vi "QR_registro_testcompleto.vi"() -> ()   [LabVIEW 2019]
uses:
  <vilib>/Instr/_visa.llb/VISA Configure Serial Port (Instr).vi
  <vilib>/regexp/Match Regular Expression.xnode
panel:
  in  "?":bool
  out "Boolean":bool
  in  "Cerrar socket":bool
  in  "Abrir socket":bool
  out "Error_QR":bool
  in  "Interruptor Error":bool
  in  "stop socket 2":bool
  out "Bytes at port 3":u32=1
  in  "IN y":string(combo)="00"
  in  "IN x":string(combo)="00"
  in  "NOK y":string(combo)="00"
  in  "NOK x":string(combo)="00"
  in  "OK y":string(combo)="00"
  in  "OK x":string(combo)="00"
  in  "Operator's name":string(combo)="Juan Rodríguez"
  in  "?":bool
  in  "Fichero de registro":path=path "C:/Trabajo_Robot/desde Marzo 2023/Pruebas_PC_APD/RESULT_TEST_C_LABP0"
  in  "Config File":path=path "C:/Trabajo/Test Asic Javi_2021/Origen Socket SERVO_PCB_BUENO_v5 (muchos asics)/CONFIG/configuracion_robot_CTAV2022A.test"
  in  "Path Out Report":path=path "C:/Trabajo_Robot/desde Marzo 2023/Pruebas_PC_APD/RESULT_TEST_C_LABP0"
  out "Datos_QR":string
  in  "stop socket":bool
  out "Bytes at port 1":u32
  in  "Enviar":bool
  out "Iteraciones":i32=1
  out "Lectura buffer":string="1"
  in  "Delay (ms)":dbl=1.0 min=1.0 max=9.0 step=1.0
  out "Bytes at port 2":u32=1
  out "message":string=" INSTRUCTIONS:\r\rNormal Use:  When using subVIs that incorporate the error in/error out (or error I/O) structure, place this handler where you want to inform the user of an error, typically at the end of the I/O data path, as the last action of the program.  If the error in error? is ERROR, the handler creates a message describing the error and its source.  If the type of dialog = 1 (default), the message is displayed to the user, who can only acknowedge it.  If the type = 2, the user can acknowledge the message or abort execution; aborting a program with active I/O is not recommended.  If the type = 0, no message is displayed; this is used to process the error programmatically, and the error out cluster elements are wired to individual terminals for that reason.  \r\rOther Use:\n\r\nlocal testing.  To test the error code of a subVI or function that does not have the error I/O structure, you can wire its error code and a source string to the local error code and error source inputs.  If error in error? indicates no error and error code is not equal to 0, the local code and source are substituted for the error in values, and error? is set TRUE (ERROR)."
  in  "Interruptor":bool
  in  "stop":bool
  # "Funcionamiento: en la primera iteración, el efector se desplaza desde el origen hasta la celda\nintroducida, hace una pausa, va a la posición del socket (0,0), hace otra pausa, va a la celda\nde salida y vuelve al origen. En las iteraciones siguientes hará lo mismo pero recorriendo las\nceldas de la bandeja sucesivamente. Que el desplazamiento se produzca hacia una celda de\nla bandeja OK o de la bandeja NOK depende de la salidad del programa de test de Asics."
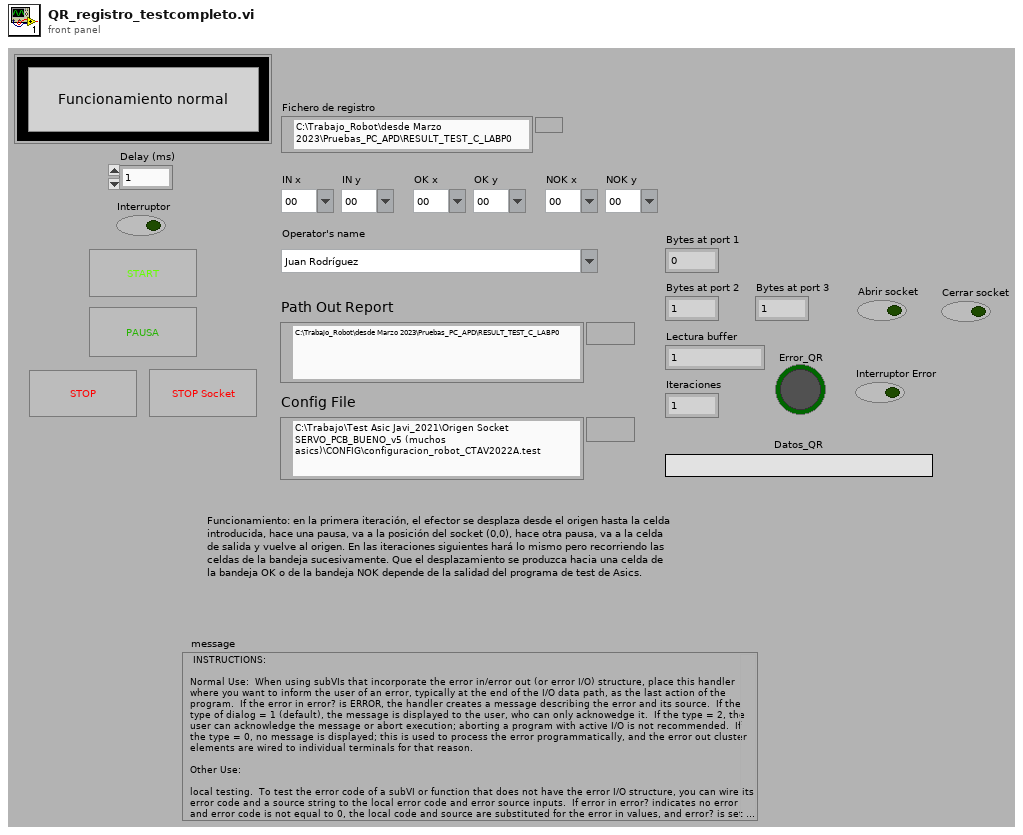
[diagram p1: front panel]
types:
  T1 = enum16{"open", "replace", "create", "open or create", "replace or create", "replace or create with confirmation"}
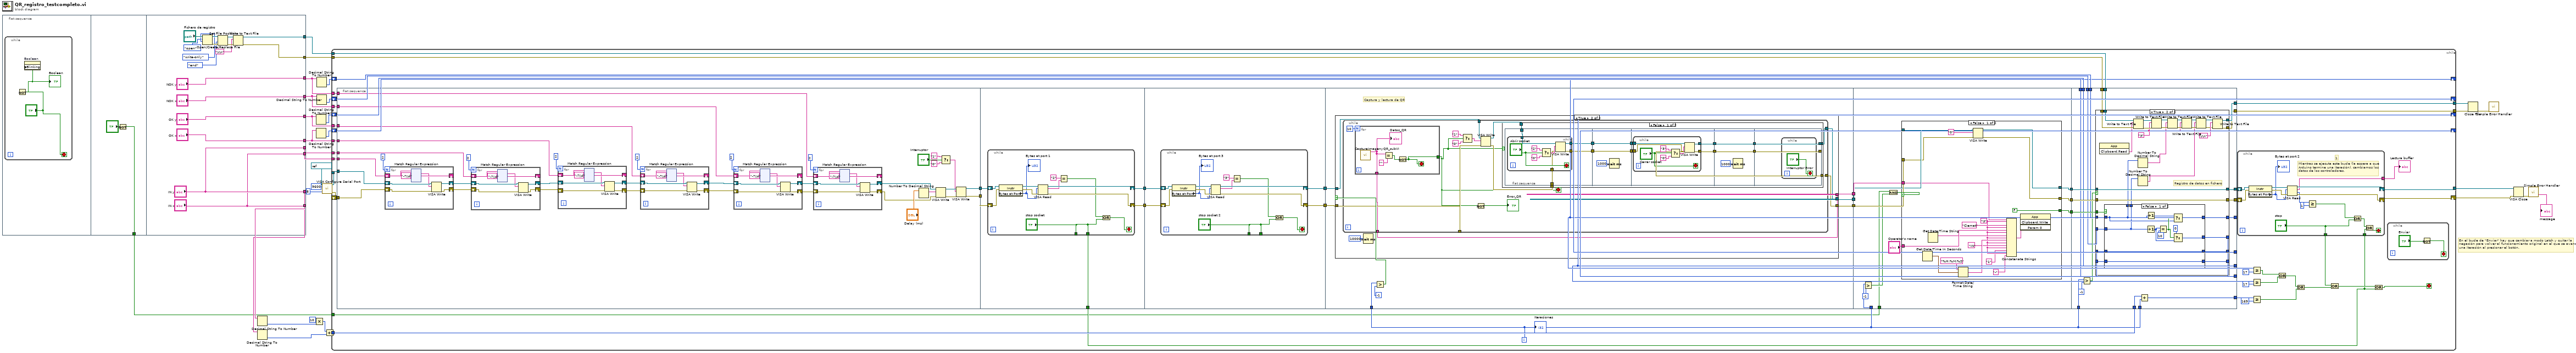
[diagram p0: block diagram]
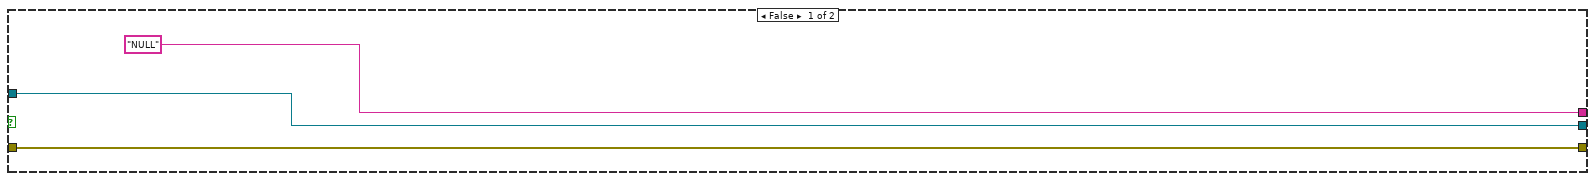
[diagram p2: hidden frame]
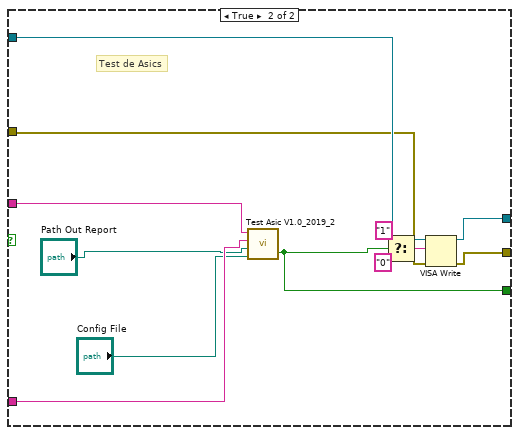
[diagram p4: hidden frame]
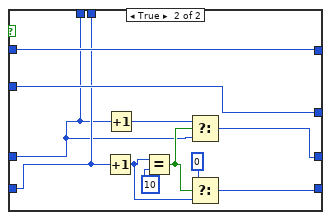
[diagram p6: hidden frame]
diagram:
  # "En el bucle de \"Enviar\" hay que cambiar a modo Latch y quitar la\nnegación para volver al funcionamiento original en el que se avanza\nuna iteración al presionar el botón."
  n1 = flat-sequence {
    tunnel: [w35] -> w1
    tunnel: ["NOK y"] -> w16
    tunnel: ["NOK x"] -> w15
    tunnel: ["OK y"] -> w14
    tunnel: ["OK x"] -> w13
    tunnel: ["IN y"] -> w12
    tunnel: ["IN x"] -> w11
    tunnel: [w37] -> w10
    tunnel: [w38] -> w9
    tunnel: ["IN y"] -> w8
    tunnel: ["IN x"] -> w7
    frame #0 {
      n2 = while {
        stop <- "?" stop-if-true
        n3 = Not(x="?") -> (.not. x?=w33:bool)
        "Boolean" <- w33
        n4 = property on="Boolean" class="Bool (strict)"("Blinking"=w33) -> ()  [unwired: 2 in, 2 out]
      }
    }
    frame #1 {
      n5 = Not(x="?") -> (.not. x?=w35:bool)
    }
    frame #2 {
      n6 = Open/Create/Replace File(file path (use dialog)="Fichero de registro", operation (0:open)=T1."open", access (0:read/write)=enum16{"read/write", "read-only", "write-only"}."write-only") -> (refnum out=w49:refnum<file>, error out=w52:errorcluster)  [unwired: 3 in, 1 out]
      n7 = Set File Position(refnum=w49, from (0:start)=enum16{"start", "end", "current"}."end", error in=w52) -> (refnum out=w50:refnum<file>, error out=w53:errorcluster)  [unwired: 1 in]
      n8 = Write to Text File(file (use dialog)=w50, text="\r\n", error in=w53) -> (refnum out=w38:refnum<file>, error out=w37:errorcluster)  [unwired: 1 in, 1 out]
    }
  }
  n9 = Decimal String To Number(string=w8) -> (number=w6:i32)  [unwired: 2 in, 1 out]
  n10 = Decimal String To Number(string=w7) -> (number=w3:i32)  [unwired: 2 in, 1 out]
  n11 = Multiply(x=10, y=w6) -> (x*y=w4:i32)
  n12 = Decimal String To Number(string=w14) -> (number=w18:i32)  [unwired: 2 in, 1 out]
  n13 = Decimal String To Number(string=w13) -> (number=w17:i32)  [unwired: 2 in, 1 out]
  n14 = Decimal String To Number(string=w16) -> (number=w20:i32)  [unwired: 2 in, 1 out]
  n15 = Decimal String To Number(string=w15) -> (number=w19:i32)  [unwired: 2 in, 1 out]
  n16 = call-poly "VISA Configure Serial Port"("VISA resource name"=refnum<visa-resource-name> "COM9", "baud rate (9600)"=u32 9600, "data bits (8)"=u16 8) -> ("VISA resource name out"=w24:refnum<visa-resource-name>, "error out"=w27:errorcluster)  [unwired: 11 in]
  n17 = Add(x=w4, y=w3) -> (x+y=w2:i32)
  n18 = while {
    shift-right: [w104] -> w25
    shift-left: w27 -> [w106]
    tunnel: w24 -> [w102]
    tunnel: [w105] -> w26
    tunnel: w9 -> [w95]
    tunnel: [w94] -> w23
    tunnel: w10 -> [w93]
    tunnel: [w92] -> w22
    tunnel: w11 -> [w90]
    tunnel: w12 -> [w89]
    tunnel: w13 -> [w88]
    tunnel: w14 -> [w87]
    tunnel: w15 -> [w86]
    tunnel: w16 -> [w85]
    shift-right: [w78] -> _
    shift-left: w20 -> [w84]
    shift-right: [w80] -> _
    shift-left: w19 -> [w83]
    shift-right: [w76] -> _
    shift-left: w18 -> [w82]
    shift-right: [w79] -> _
    shift-left: w17 -> [w81]
    tunnel: w2 -> [w72]
    tunnel: w1 -> [w54]
    i -> [w55]
    stop <- w64 stop-if-true
    n19 = flat-sequence {
      tunnel: w106 -> [w142]
      tunnel: w102 -> [w131]
      tunnel: [w133] -> w101
      tunnel: [w132] -> w100
      tunnel: w90 -> [w112]
      tunnel: w89 -> [w111]
      tunnel: w88 -> [w110]
      tunnel: w87 -> [w109]
      tunnel: w86 -> [w108]
      tunnel: w85 -> [w107]
      tunnel: w101 -> [w879]
      tunnel: w100 -> [w878]
      tunnel: [w877] -> w62
      tunnel: [w876] -> w60
      tunnel: [w875] -> w63
      tunnel: w62 -> [w895]
      tunnel: [w893] -> w61
      tunnel: w60 -> [w894]
      tunnel: [w892] -> w59
      tunnel: w61 -> [w913]
      tunnel: w59 -> [w912]
      tunnel: w55 -> [w914]
      tunnel: [w910] -> w58
      tunnel: [w909] -> w57
      tunnel: [w908] -> w56
      tunnel: w55 -> [w998]
      tunnel: [w1000] -> w98
      tunnel: [w999] -> w97
      tunnel: [w996] -> w91
      tunnel: w58 -> [w995]
      tunnel: w57 -> [w994]
      tunnel: w56 -> [w993]
      tunnel: w54 -> [w990]
      tunnel: [w1047] -> w96
      tunnel: [w1049] -> w99
      tunnel: w98 -> [w1048]
      tunnel: w97 -> [w1046]
      tunnel: w95 -> [w1053]
      tunnel: [w1052] -> w94
      tunnel: w93 -> [w1051]
      tunnel: [w1050] -> w92
      tunnel: w55 -> [w1043]
      tunnel: w91 -> [w1042]
      tunnel: w84 -> [w1038]
      tunnel: w83 -> [w1041]
      tunnel: w82 -> [w1040]
      tunnel: w81 -> [w1039]
      tunnel: [w1037] -> w78
      tunnel: [w1036] -> w80
      tunnel: [w1035] -> w76
      tunnel: [w1034] -> w79
      tunnel: w72 -> [w1033]
      tunnel: w55 -> [w1032]
      tunnel: [w1031] -> w71
      frame #0 {
        n20 = for {
          N: 2 -> [_]
          shift-right: [w754] -> _
          shift-left: w112 -> [w759]
          shift-right: [w757] -> w128
          shift-left: w131 -> [w758]
          shift-right: [w755] -> w127
          shift-left: w142 -> [w756]
          n21 = xnode "Match Regular Expression"("input string"=w759, "regular expression"="-?\\d") -> ("whole match"=w753:string, "after match"=w754:string)  [unwired: 4 in, 3 out]
          n22 = VISA Write(VISA resource name=w758, write buffer=w753, error in (no error)=w756) -> (VISA resource name out=w757:refnum<visa-resource-name>, error out=w755:errorcluster)  [unwired: 1 out]
        }
        n23 = for {
          N: 2 -> [_]
          shift-right: [w632] -> _
          shift-left: w111 -> [w637]
          shift-right: [w635] -> w122
          shift-left: w128 -> [w636]
          shift-right: [w633] -> w121
          shift-left: w127 -> [w634]
          n24 = xnode "Match Regular Expression"("input string"=w637, "regular expression"="-?\\d") -> ("whole match"=w631:string, "after match"=w632:string)  [unwired: 4 in, 3 out]
          n25 = VISA Write(VISA resource name=w636, write buffer=w631, error in (no error)=w634) -> (VISA resource name out=w635:refnum<visa-resource-name>, error out=w633:errorcluster)  [unwired: 1 out]
        }
        n26 = for {
          N: 2 -> [_]
          shift-right: [w510] -> _
          shift-left: w110 -> [w515]
          shift-right: [w513] -> w124
          shift-left: w122 -> [w514]
          shift-right: [w511] -> w123
          shift-left: w121 -> [w512]
          n27 = xnode "Match Regular Expression"("input string"=w515, "regular expression"="-?\\d") -> ("whole match"=w509:string, "after match"=w510:string)  [unwired: 4 in, 3 out]
          n28 = VISA Write(VISA resource name=w514, write buffer=w509, error in (no error)=w512) -> (VISA resource name out=w513:refnum<visa-resource-name>, error out=w511:errorcluster)  [unwired: 1 out]
        }
        n29 = for {
          N: 2 -> [_]
          shift-right: [w388] -> _
          shift-left: w109 -> [w393]
          shift-right: [w391] -> w116
          shift-left: w124 -> [w392]
          shift-right: [w389] -> w115
          shift-left: w123 -> [w390]
          n30 = xnode "Match Regular Expression"("input string"=w393, "regular expression"="-?\\d") -> ("whole match"=w387:string, "after match"=w388:string)  [unwired: 4 in, 3 out]
          n31 = VISA Write(VISA resource name=w392, write buffer=w387, error in (no error)=w390) -> (VISA resource name out=w391:refnum<visa-resource-name>, error out=w389:errorcluster)  [unwired: 1 out]
        }
        n32 = for {
          N: 2 -> [_]
          shift-right: [w266] -> _
          shift-left: w108 -> [w271]
          shift-right: [w269] -> w118
          shift-left: w116 -> [w270]
          shift-right: [w267] -> w117
          shift-left: w115 -> [w268]
          n33 = xnode "Match Regular Expression"("input string"=w271, "regular expression"="-?\\d") -> ("whole match"=w265:string, "after match"=w266:string)  [unwired: 4 in, 3 out]
          n34 = VISA Write(VISA resource name=w270, write buffer=w265, error in (no error)=w268) -> (VISA resource name out=w269:refnum<visa-resource-name>, error out=w267:errorcluster)  [unwired: 1 out]
        }
        n35 = for {
          N: 2 -> [_]
          shift-right: [w144] -> _
          shift-left: w107 -> [w149]
          shift-right: [w147] -> w114
          shift-left: w118 -> [w148]
          shift-right: [w145] -> w113
          shift-left: w117 -> [w146]
          n36 = xnode "Match Regular Expression"("input string"=w149, "regular expression"="-?\\d") -> ("whole match"=w143:string, "after match"=w144:string)  [unwired: 4 in, 3 out]
          n37 = VISA Write(VISA resource name=w148, write buffer=w143, error in (no error)=w146) -> (VISA resource name out=w147:refnum<visa-resource-name>, error out=w145:errorcluster)  [unwired: 1 out]
        }
        n38 = Number To Decimal String(number="Delay (ms)") -> (decimal integer string=w136:string)  [unwired: 1 in]
        n39 = VISA Write(VISA resource name=w114, write buffer=w136, error in (no error)=w113) -> (VISA resource name out=w138:refnum<visa-resource-name>, error out=w137:errorcluster)  [unwired: 1 out]
        n40 = Select(t="1" ("write buffer"), s="Interruptor", f="0" ("write buffer")) -> (s? t:f=w134:string)
        n41 = VISA Write(VISA resource name=w138, write buffer=w134, error in (no error)=w137) -> (VISA resource name out=w133:refnum<visa-resource-name>, error out=w132:errorcluster)  [unwired: 1 out]
      }
      frame #1 {
        n42 = while {
          shift-right: [w885] -> w876
          shift-left: w878 -> [w890]
          tunnel: ["stop socket"] -> _
          shift-right: [w886] -> w877
          shift-left: w879 -> [w891]
          tunnel: ["stop socket"] -> w875
          stop <- w881 stop-if-true
          n43 = property class="Instr"(reference=w891, error in=w890) -> (reference out=w889:refnum<visa-resource-name>, error out=w888:errorcluster, "Bytes at Port"=w887:u32)
          "Bytes at port 1" <- w887
          n44 = VISA Read(VISA resource name=w889, byte count=w887, error in (no error)=w888) -> (VISA resource name out=w886:refnum<visa-resource-name>, read buffer=w884:string, error out=w885:errorcluster)  [unwired: 1 out]
          n45 = Equal?(x="2", y=w884) -> (x = y?=w882:bool)
          n46 = Or(x=w882, y="stop socket") -> (x .or. y?=w881:bool)
        }
      }
      frame #2 {
        n47 = while {
          shift-right: [w901] -> w892
          shift-left: w894 -> [w906]
          tunnel: ["stop socket 2"] -> _
          shift-right: [w902] -> w893
          shift-left: w895 -> [w907]
          tunnel: ["stop socket 2"] -> _
          stop <- w897 stop-if-true
          n48 = property class="Instr"(reference=w907, error in=w906) -> (reference out=w905:refnum<visa-resource-name>, error out=w904:errorcluster, "Bytes at Port"=w903:u32)
          "Bytes at port 3" <- w903
          n49 = VISA Read(VISA resource name=w905, byte count=w903, error in (no error)=w904) -> (VISA resource name out=w902:refnum<visa-resource-name>, read buffer=w900:string, error out=w901:errorcluster)  [unwired: 1 out]
          n50 = Equal?(x="3", y=w900) -> (x = y?=w898:bool)
          n51 = Or(x=w898, y="stop socket 2") -> (x .or. y?=w897:bool)
        }
      }
      frame #3 {
        # "Captura y lectura de QR"
        n52 = Greater?(x=w914, y=-1) -> (0:w911:bool)
        n53 = case shown="True" w911 {
          tunnel: [w918 w921] -> w908
          tunnel: w913 -> [w918 w922]
          tunnel: [w917 w920] -> w910
          tunnel: w912 -> [w917 w919]
          tunnel: ["NULL" ("Datos_QR") w923] -> w909
          frame False {
          }
          frame True {
            n54 = while {
              tunnel: [w937] -> w923
              tunnel: w922 -> [w935]
              tunnel: [w931] -> w921
              tunnel: [w930] -> w920
              tunnel: w919 -> [w928]
              stop <- w925 stop-if-true
              n55 = for {
                N: 10 -> [_]
                tunnel: [w987] -> w937
                tunnel: [w985] -> w925
                stop <- w985 stop-if-true
                n56 = call "CapturaImagenyQR_subVI.vi"() -> ("Datos_QR"=w987:string)  [unwired: 11 in]
                "Datos_QR" <- w987
                n57 = Equal?(x=w987, y="" ("Datos_QR")) -> (x = y?=w986:bool)
                n58 = Not(x=w986) -> (.not. x?=w985:bool)
              }
              n59 = Select(t="1" ("write buffer"), s=w925, f="0" ("write buffer")) -> (s? t:f=w932:string)
              n60 = Not(x=w925) -> (.not. x?=→"Error_QR":bool)
              n61 = VISA Write(VISA resource name=w935, write buffer=w932, error in (no error)=w928) -> (VISA resource name out=w929:refnum<visa-resource-name>, error out=w927:errorcluster)  [unwired: 1 out]
              n62 = case shown="False" w925 {
                tunnel: w929 -> [w949 w984]
                tunnel: w927 -> [w948 w983]
                tunnel: [w947 w984] -> w931
                tunnel: [w946 w983] -> w930
                frame False {
                  n63 = flat-sequence {
                    tunnel: w949 -> [w953]
                    tunnel: [w952] -> w945
                    tunnel: [w951] -> w943
                    tunnel: w948 -> [w950]
                    tunnel: w945 -> [w964]
                    tunnel: [w964] -> w944
                    tunnel: w943 -> [w963]
                    tunnel: [w963] -> w942
                    tunnel: w944 -> [w968]
                    tunnel: w942 -> [w967]
                    tunnel: [w966] -> w941
                    tunnel: [w965] -> w939
                    tunnel: w941 -> [w979]
                    tunnel: [w979] -> w940
                    tunnel: w939 -> [w978]
                    tunnel: [w978] -> w938
                    tunnel: [w980] -> w946
                    tunnel: [w981] -> w947
                    tunnel: w940 -> [w981]
                    tunnel: w938 -> [w980]
                    frame #0 {
                      n64 = while {
                        tunnel: w953 -> [w961]
                        tunnel: [w956] -> w952
                        tunnel: [w955] -> w951
                        tunnel: w950 -> [w954]
                        stop <- "Abrir socket" stop-if-true
                        n65 = Select(t="2" ("write buffer"), s="Abrir socket", f="0" ("write buffer")) -> (s? t:f=w958:string)
                        n66 = VISA Write(VISA resource name=w961, write buffer=w958, error in (no error)=w954) -> (VISA resource name out=w956:refnum<visa-resource-name>, error out=w955:errorcluster)  [unwired: 1 out]
                      }
                    }
                    frame #1 {
                      n67 = Wait (ms)(milliseconds to wait=u32 1000) -> ()  [unwired: 1 out]
                    }
                    frame #2 {
                      n68 = while {
                        tunnel: w968 -> [w972]
                        tunnel: w967 -> [w971]
                        tunnel: [w970] -> w966
                        tunnel: [w969] -> w965
                        stop <- "Cerrar socket" stop-if-true
                        n69 = Select(t="3" ("write buffer"), s="Cerrar socket", f="0" ("write buffer")) -> (s? t:f=w974:string)
                        n70 = VISA Write(VISA resource name=w972, write buffer=w974, error in (no error)=w971) -> (VISA resource name out=w970:refnum<visa-resource-name>, error out=w969:errorcluster)  [unwired: 1 out]
                      }
                    }
                    frame #3 {
                      n71 = Wait (ms)(milliseconds to wait=u32 1000) -> ()  [unwired: 1 out]
                    }
                    frame #4 {
                      n72 = while {
                        stop <- "Interruptor Error" stop-if-true
                      }
                    }
                  }
                }
                frame True {
                }
              }
            }
            n73 = Wait (ms)(milliseconds to wait=u32 10000) -> ()  [unwired: 1 out]
          }
        }
      }
      frame #4 {
        n74 = Greater?(x=w998, y=-1) -> (0:w992:bool)
        n75 = And(x=w990, y=w992) -> (x .and. y?=w991:bool)
        n76 = case shown="False" w991 {
          tunnel: w993 -> [w1016 w1027]
          tunnel: w995 -> [w1015 w1026]
          tunnel: [w1014 w1025] -> w1000
          tunnel: [w1013 w1024] -> w999
          tunnel: w994 -> [w1009 w1023]
          tunnel: [FALSE ("Boolean") w1019] -> w996
          tunnel: "Operator's name" -> [w1007 w1022]
          frame False {
            w1003 = "\t"
            n77 = Get Date/Time In Seconds() -> (seconds since 1Jan1904=w1011:timestamp)
            n78 = Get Date/Time String() -> (date string=w1006:string)  [unwired: 3 in, 1 out]
            n79 = Format Date/Time String(time format string (%c)="%H:%M:%S", seconds (now)=w1011) -> (date/time string=w1005:string)  [unwired: 1 in]
            n80 = VISA Write(VISA resource name=w1016, write buffer="0", error in (no error)=w1015) -> (VISA resource name out=w1014:refnum<visa-resource-name>, error out=w1013:errorcluster)  [unwired: 1 out]
            n81 = Concatenate Strings(w1009, w1003, "Ciemat", w1003, w1007, w1003, w1006, w1003, w1005, w1003, "IN", w1003, "1", w1003, "-") -> (w1012:string)
            n82 = invoke class="App" method="Clipboard.Write"("Param 0"=w1012) -> ()  [unwired: 3 in, 4 out]
          }
          frame True {
            # "Test de Asics"
            n83 = call "Test Asic V1.0_2019_2.vi"("Config File"="Config File", "Path Out Report"="Path Out Report", "Operator's Name"=w1022, "ASIC'S Number"=w1023) -> ("OK, Fault 2"=w1019:bool)  [unwired: 1 in]
            n84 = Select(t="1" ("write buffer"), s=w1019, f="0" ("write buffer")) -> (s? t:f=w1028:string)
            n85 = VISA Write(VISA resource name=w1027, write buffer=w1028, error in (no error)=w1026) -> (VISA resource name out=w1025:refnum<visa-resource-name>, error out=w1024:errorcluster)  [unwired: 1 out]
          }
        }
      }
      frame #5 {
        n86 = Greater?(x=w1043, y=-1) -> (0:w1044:bool)
        n87 = case shown="True" w1044 {
          tunnel: w1053 -> [w1059 w1092]
          tunnel: [w1059 w1091] -> w1052
          tunnel: w1051 -> [w1058 w1090]
          tunnel: [w1058 w1089] -> w1050
          tunnel: [w1061 w1088] -> w1049
          tunnel: w1048 -> [w1061 w1088]
          tunnel: [w1060 w1087] -> w1047
          tunnel: w1046 -> [w1060 w1087]
          tunnel: w1042 -> [_ w1085]
          tunnel: w1038 -> [w1057 w1084]
          tunnel: w1041 -> [w1056 w1083]
          tunnel: w1040 -> [w1055 w1082]
          tunnel: w1039 -> [w1054 w1081]
          tunnel: [w1057 w1080] -> w1037
          tunnel: [w1056 w1079] -> w1036
          tunnel: [w1055 w1078] -> w1035
          tunnel: [w1054 w1077] -> w1034
          frame False {
          }
          frame True {
            w1064 = "\t"
            # "Registro de datos en fichero"
            n88 = invoke class="App" method="Clipboard.Read"() -> ("Read Clipbrd"=w1086:string)  [unwired: 3 in, 2 out]
            n89 = case shown="False" w1085 {
              tunnel: w1084 -> [w1095 w1108]
              tunnel: w1083 -> [w1094 w1107]
              tunnel: w1082 -> [w1097 w1105]
              tunnel: w1081 -> [w1096 w1106]
              tunnel: [w1099 w1108] -> w1080
              tunnel: [w1098 w1107] -> w1079
              tunnel: [w1097 w1110] -> w1078
              tunnel: [w1096 w1109] -> w1077
              tunnel: [w1095 w1105] -> w1076
              tunnel: [w1094 w1106] -> w1075
              frame False {
                n90 = Increment(x=w1094) -> (x+1=w1103:i32)
                n91 = Increment(x=w1095) -> (x+1=w1100:i32)
                n92 = Equal?(x=w1103, y=10) -> (x = y?=w1101:bool)
                n93 = Select(t=w1100, s=w1101, f=w1095) -> (s? t:f=w1099:i32)
                n94 = Select(t=0, s=w1101, f=w1103) -> (s? t:f=w1098:i32)
              }
              frame True {
                n95 = Increment(x=w1106) -> (x+1=w1114:i32)
                n96 = Increment(x=w1105) -> (x+1=w1111:i32)
                n97 = Equal?(x=w1114, y=10) -> (x = y?=w1112:bool)
                n98 = Select(t=w1111, s=w1112, f=w1105) -> (s? t:f=w1110:i32)
                n99 = Select(t=0, s=w1112, f=w1114) -> (s? t:f=w1109:i32)
              }
            }
            n100 = Write to Text File(file (use dialog)=w1092, text=w1086, error in=w1090) -> (refnum out=w1073:refnum<file>, error out=w1074:errorcluster)  [unwired: 1 in, 1 out]
            n101 = Number To Decimal String(number=w1076) -> (decimal integer string=w1063:string)  [unwired: 1 in]
            n102 = Number To Decimal String(number=w1075) -> (decimal integer string=w1062:string)  [unwired: 1 in]
            n103 = Write to Text File(file (use dialog)=w1073, text=w1064, error in=w1074) -> (refnum out=w1071:refnum<file>, error out=w1072:errorcluster)  [unwired: 1 in, 1 out]
            n104 = Write to Text File(file (use dialog)=w1071, text=w1063, error in=w1072) -> (refnum out=w1068:refnum<file>, error out=w1067:errorcluster)  [unwired: 1 in, 1 out]
            n105 = Write to Text File(file (use dialog)=w1068, text=w1064, error in=w1067) -> (refnum out=w1066:refnum<file>, error out=w1065:errorcluster)  [unwired: 1 in, 1 out]
            n106 = Write to Text File(file (use dialog)=w1066, text=w1062, error in=w1065) -> (refnum out=w1070:refnum<file>, error out=w1069:errorcluster)  [unwired: 1 in, 1 out]
            n107 = Write to Text File(file (use dialog)=w1070, text="\r\n", error in=w1069) -> (refnum out=w1091:refnum<file>, error out=w1089:errorcluster)  [unwired: 1 in, 1 out]
          }
        }
        n108 = Add(x=w1033, y=w1032) -> (x+y=w1031:i32)
      }
    }
    n109 = while {
      shift-right: [w1125] -> w104
      shift-left: w96 -> [w1131]
      tunnel: ["stop"] -> w66
      shift-right: [w1126] -> w105
      shift-left: w99 -> [w1132]
      tunnel: [w1121] -> w103
      tunnel: w63 -> [w1118]
      stop <- w1120 stop-if-true
      # "1"
      # "Mientras se ejecuta este bucle (la espera a que\nArduino termine una iteración), cambiamos los\ndatos de los controladores."
      n110 = property class="Instr"(reference=w1132, error in=w1131) -> (reference out=w1129:refnum<visa-resource-name>, error out=w1128:errorcluster, "Bytes at Port"=w1127:u32)
      "Bytes at port 2" <- w1127
      n111 = VISA Read(VISA resource name=w1129, byte count=w1127, error in (no error)=w1128) -> (VISA resource name out=w1126:refnum<visa-resource-name>, read buffer=w1121:string, return count=w1124:u32, error out=w1125:errorcluster)
      n112 = Greater Or Equal?(x=w1124, y=u32 1) -> (x >= y?=w1122:bool)
      n113 = Or(x=w1122, y="stop") -> (x .or. y?=w1119:bool)
      n114 = Or(x=w1119, y=w1118) -> (x .or. y?=w1120:bool)
    }
    "Lectura buffer" <- w103
    n115 = Greater Or Equal?(x=w78, y=17) -> (x >= y?=w74:bool)
    n116 = Greater Or Equal?(x=w76, y=17) -> (x >= y?=w73:bool)
    n117 = Greater Or Equal?(x=w71, y=169) -> (x >= y?=w69:bool)
    n118 = Or(x=w74, y=w73) -> (x .or. y?=w68:bool)
    n119 = Or(x=w68, y=w69) -> (x .or. y?=w67:bool)
    n120 = Or(x=w66, y=w67) -> (x .or. y?=w65:bool)
    n121 = Or(x=w65, y=w63) -> (x .or. y?=w64:bool)
    n122 = while {
      stop <- w1116 stop-if-true
      n123 = Not(x="Enviar") -> (.not. x?=w1116:bool)
    }
    "Iteraciones" <- w55
  }
  n124 = Close File(refnum=w23, error in=w22) -> (error out=w21:errorcluster)  [unwired: 1 out]
  n125 = call <vilib>:"Simple Error Handler.vi"("error in (no error)"=w21) -> ()  [unwired: 4 in, 5 out]
  n126 = VISA Close(VISA resource name=w26, error in (no error)=w25) -> (error out=w31:errorcluster)
  n127 = call <vilib>:"Simple Error Handler.vi"("error in (no error)"=w31) -> ("message"=→"message":string)  [unwired: 4 in, 4 out]
